vi "For_DoWhile_Timer.vi"() -> ()   [LabVIEW 2015]
panel:
  out "Numeric 2":dbl
  in  "stop":bool
  out "Array":i32[](array[numeric])
  in  "Numeric":i32
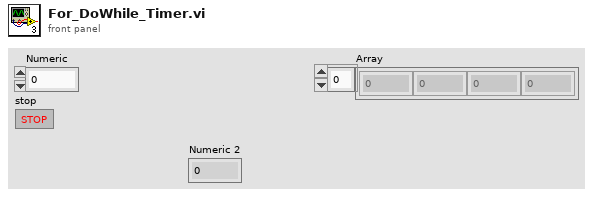
[diagram p1: front panel]
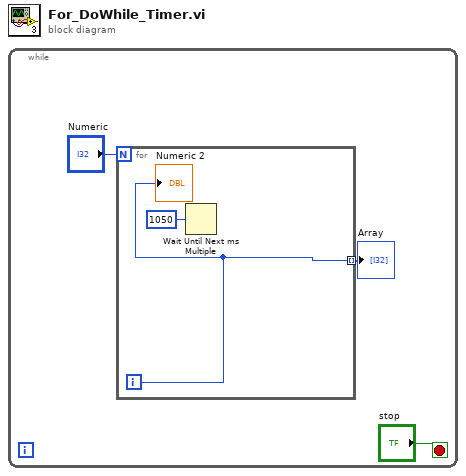
[diagram p0: block diagram]
diagram:
  n1 = while {
    stop <- "stop" stop-if-true
    n2 = for {
      N: "Numeric" -> [_]
      tunnel: [w4] -> w2 mode=indexing
      i -> [w4]
      n3 = Wait Until Next ms Multiple(millisecond multiple=u32 1050) -> ()  [unwired: 1 out]
      "Numeric 2" <- w4
    }
    "Array" <- w2
  }
